vi "sub.vi"(11 "arguments":T1[](array[typedef])) -> (3 "Expression":T1)   [LabVIEW 2021]
uses:
  Expression.ctl
  ExpressionType.ctl
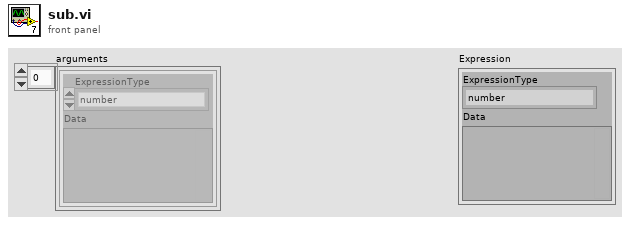
[diagram p1: front panel]
types:
  T1 = typedef "Expression.ctl" = cluster{"ExpressionType":T2, "Data":variant}
  T2 = typedef "ExpressionType.ctl" = enum16{"number", "string", "symbol", "primitive", "list", "closure", "nil", "error"}
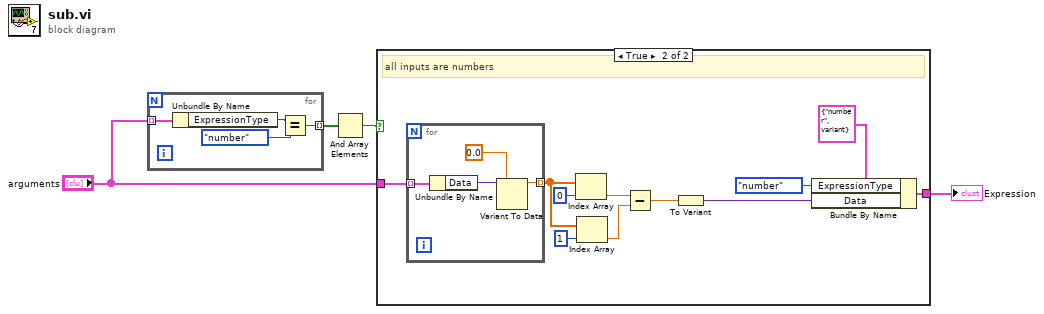
[diagram p0: block diagram]
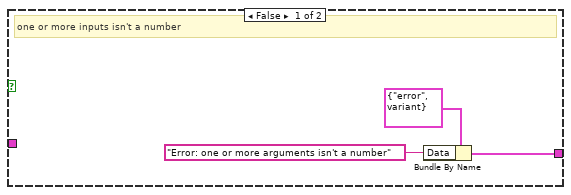
[diagram p2: hidden frame]
diagram:
  n1 = for {
    tunnel: "arguments" -> [w8] mode=indexing
    tunnel: [w5] -> w3 mode=indexing
    n2 = Unbundle By Name(w8) -> ("ExpressionType"=w7:T2)
    n3 = Equal?(x=w7, y=ExpressionType."number") -> (x = y?=w5:bool)
  }
  n4 = And Array Elements(Boolean array=w3) -> (logical AND=w2:bool)
  n5 = case shown="True" w2 {
    tunnel: [w9 w20] -> w4
    tunnel: "arguments" -> [_ w18]
    frame False {
      # "one or more inputs isn't a number"
      n6 = Bundle By Name(cluster=T1 {"ExpressionType"=enum."error", "Data"=variant} ("Expression 3"), "Data"="Error: one or more arguments isn't a number") -> (w9:T1)
    }
    frame True {
      # "all inputs are numbers"
      n7 = for {
        tunnel: w18 -> [w26] mode=indexing
        tunnel: [w23] -> w15 mode=indexing
        n8 = Unbundle By Name(w26) -> ("Data"=w25:variant)
        n9 = Variant To Data(type=0.0, Variant=w25) -> (data=w23:dbl)  [unwired: 1 in, 1 out]
      }
      n10 = Index Array(array=w15, index=0) -> (element=w14:dbl)
      n11 = Index Array(array=w15, index=1) -> (element=w13:dbl)
      n12 = Subtract(x=w14, y=w13) -> (x-y=w12:dbl)
      n13 = To Variant(anything=w12) -> (Variant=w19:variant)
      n14 = Bundle By Name(cluster=T1 {"ExpressionType"=enum."number", "Data"=variant} ("Expression 3"), "ExpressionType"=ExpressionType."number", "Data"=w19) -> (w20:T1)
    }
  }
  "Expression" <- w4
